vi "Read Driver Joystick.vi"   [LabVIEW 2020]
uses:
  <vilib>/Rock Robotics/WPI/Utilities/WPI_GetSetVariantRefNum.vi
  <vilib>/Rock Robotics/Network Tables/NT Write Boolean Array.vi
  <vilib>/Rock Robotics/Network Tables/NT Write Numeric Array.vi
  Framework/Robot Global Data.vi
panel:
  # "READ DRIVER JOYSTICK"
types:
  T1 = enum16{"0", "1", "2", "3", "4", "5", "6", "7", "8", "9", "10", "11"}
  T2 = typedef "WPI_JoystickDevRef.ctl" = cluster{"Device":T3}
  T3 = typedef "WPI_JoystickDeviceEnum.ctl" = enum16{"USB 0", "USB 1", "USB 2", "USB 3", "USB 4", "USB 5"}
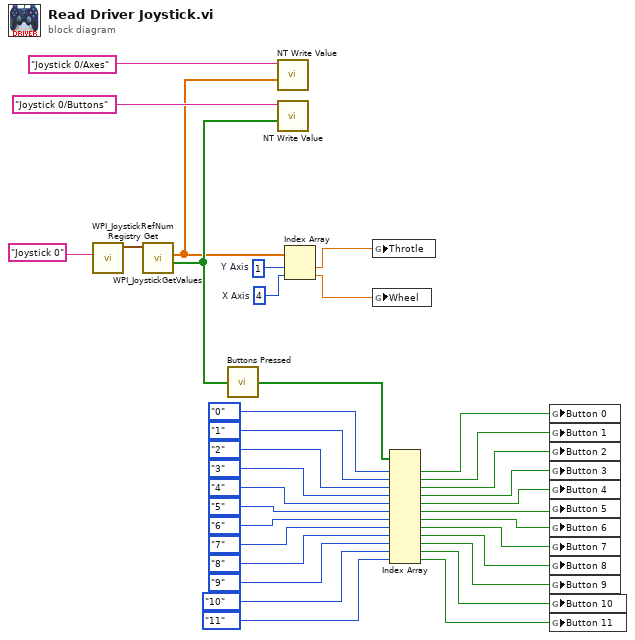
[diagram p0: block diagram]
diagram:
  w28 = 1  # Y Axis
  w27 = 4  # X Axis
  n1 = call <vilib>:"WPI_JoystickRefNum Registry Get.vi"("refnum name"="Joystick 0") -> ("JoystickDevRef"=w34:T2)  [unwired: 1 in, 9 out]
  n2 = call <vilib>:"WPI_JoystickGetValues.vi"("JoystickDevRef"=w34) -> ("Buttons"=w31:bool[], "Axes"=w30:dbl[])  [unwired: 6 in, 3 out]
  n3 = call "Buttons Pressed.vi"("Button Values"=w31) -> ("Button Presses"=w33:bool[])
  n4 = call-poly <vilib>:"NT Write Value.vi"("Numeric Array"=w30, "Name"="Joystick 0/Axes") -> ()  [unwired: 9 in, 1 out]
  n5 = call-poly <vilib>:"NT Write Value.vi"("Boolean Array"=w31, "Name"="Joystick 0/Buttons") -> ()  [unwired: 9 in, 1 out]
  n6 = Index Array(array=w30, index #1=w28, index #2=w27) -> (element #1=w14:dbl, element #2=w13:dbl)
  n7 = global write "Robot Global Data.vi" "Throtle"(w14) -> ()
  n8 = global write "Robot Global Data.vi" "Wheel"(w13) -> ()
  n9 = Index Array(array=w33, index #1=T1."0", index #2=T1."1", index #3=T1."2", index #4=T1."3", index #5=T1."4", index #6=T1."5", index #7=T1."6", index #8=T1."7", index #9=T1."8", index #10=T1."9", index #11=T1."10", index #12=T1."11") -> (element #1=w12:bool, element #2=w11:bool, element #3=w10:bool, element #4=w9:bool, element #5=w8:bool, element #6=w7:bool, element #7=w6:bool, element #8=w5:bool, element #9=w4:bool, element #10=w3:bool, element #11=w2:bool, element #12=w1:bool)
  n10 = global write "Robot Global Data.vi" "Button 0"(w12) -> ()
  n11 = global write "Robot Global Data.vi" "Button 1"(w11) -> ()
  n12 = global write "Robot Global Data.vi" "Button 2"(w10) -> ()
  n13 = global write "Robot Global Data.vi" "Button 3"(w9) -> ()
  n14 = global write "Robot Global Data.vi" "Button 4"(w8) -> ()
  n15 = global write "Robot Global Data.vi" "Button 5"(w7) -> ()
  n16 = global write "Robot Global Data.vi" "Button 6"(w6) -> ()
  n17 = global write "Robot Global Data.vi" "Button 7"(w5) -> ()
  n18 = global write "Robot Global Data.vi" "Button 8"(w4) -> ()
  n19 = global write "Robot Global Data.vi" "Button 9"(w3) -> ()
  n20 = global write "Robot Global Data.vi" "Button 10"(w2) -> ()
  n21 = global write "Robot Global Data.vi" "Button 11"(w1) -> ()
